vi "Change Blob Lease ID.vi"(4 "Proposed Lease ID":string, 6 "Current Lease ID":string, 8 "error in (no error)":errorcluster, 9 "Blob":string, 10 "Container":string, 11 "Azure Session in":refnum<class "Session.lvclass">) -> (0 "error out":errorcluster, 3 "Azure Session out":refnum<class "Session.lvclass">)   [LabVIEW 2015, in "NI_Azure_Blob.lvlib"]
doc: "Change the ID of an existing blob lease."
uses:
  NI_Azure_Blob.lvlib
  Core/Session/Session.lvclass
  Core/Name Value Pair.ctl
  Lease Action.ctl
  Core/Session/Session.lvclass/Session.ctl
  Core/Session/Write Request Headers.vi
  Core/Session/Write Request Parameters.vi
  Core/Session/Write HTTP Verb.vi
  Core/Session/Write URL Suffix.vi
  Core/NI_Azure_Core.lvlib
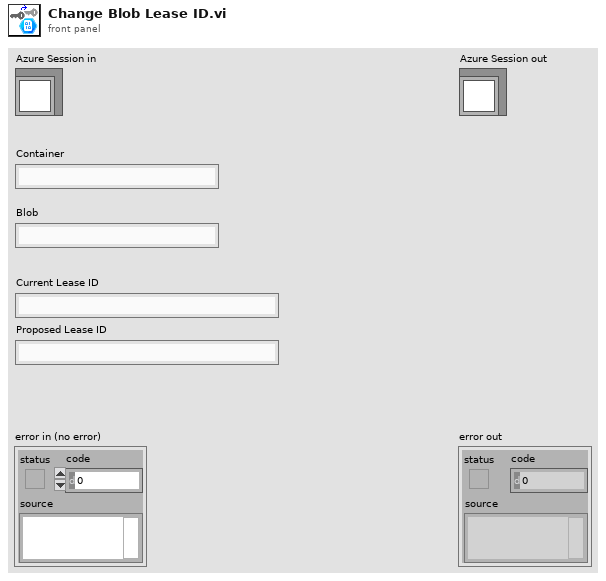
[diagram p1: front panel]
types:
  T1 = typedef "NI_Azure_Blob.lvlib/Lease Action.ctl" = enum16{"acquire", "renew", "change", "release", "break"}
  T2 = typedef "NI_Azure_Core.lvlib/Name Value Pair.ctl" = cluster{"name":string, "value":string}
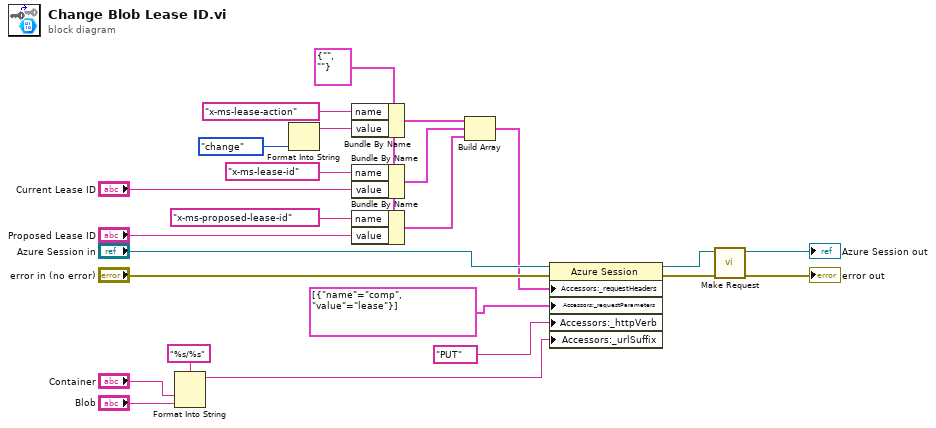
[diagram p0: block diagram]
diagram:
  w11 = T2 {"name"="", "value"=""} ("Cluster")
  n1 = Format Into String(format string="%s/%s", "Container", "Blob") -> (resulting string=w2:string)  [unwired: 2 in, 1 out]
  n2 = Format Into String(Lease_Action."change" ("Lease action")) -> (resulting string=w16:string)  [unwired: 3 in, 1 out]
  n3 = Bundle By Name(cluster=w11, "name"="x-ms-lease-action" ("header"), "value"=w16) -> (w18:T2)
  n4 = Bundle By Name(cluster=w11, "name"="x-ms-lease-id" ("header"), "value"="Current Lease ID") -> (w12:T2)
  n5 = Bundle By Name(cluster=w11, "name"="x-ms-proposed-lease-id" ("header"), "value"="Proposed Lease ID") -> (w10:T2)
  n6 = Build Array(w18, w12, w10) -> (w4:T2[])
  n7 = property class="Azure Session"(reference="Azure Session in", error in="error in (no error)", "Accessors:_requestHeaders"=w4, "Accessors:_requestParameters"=T2[] [{"name"="comp", "value"="lease"}] ("request parameters"), "Accessors:_httpVerb"="PUT" ("HTTP-Verb"), "Accessors:_urlSuffix"=w2) -> (reference out=w5:refnum<class "Session.lvclass">, error out=w7:errorcluster)
  n8 = call "Make Request.vi"("error in (no error)"=w7, "Session in"=w5) -> ("error out"=→"error out":errorcluster, "Session out"=→"Azure Session out":refnum<class "Session.lvclass">)  [unwired: 7 in, 1 out]
